vi "test_libssh2_hostkey_hash.vi"() -> ()   [LabVIEW 2017, in "integration_tests.lvlib"]
uses:
  integration_tests.lvlib
  libssh2/Host Key Hash Type.ctl
  support/support.lvlib
  libssh2/libssh2.lvlib
  <vilib>/PNR/Transparent Assertions/Transparent Assertions/Transparent Assertions.lvlib
panel:
  out "error out":errorcluster
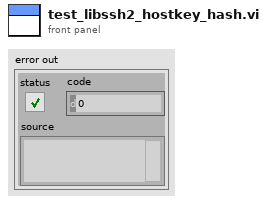
[diagram p1: front panel]
types:
  T1 = typedef "libssh2.lvlib/Host Key Hash Type.ctl" = enum16{"MD5", "SHA1", "SHA256"}
  T2 = typedef "libssh2.lvlib/Session Refnum.ctl" = refnum<k1>
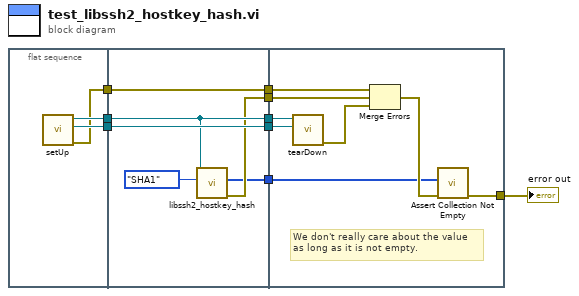
[diagram p0: block diagram]
diagram:
  n1 = flat-sequence {
    tunnel: [w12] -> w9
    tunnel: [w11] -> w8
    tunnel: [w10] -> w7
    tunnel: w9 -> [w15]
    tunnel: w8 -> [w18]
    tunnel: [w15] -> w6
    tunnel: [w18] -> w5
    tunnel: w7 -> [w17]
    tunnel: [w17] -> w4
    tunnel: [w14] -> w3
    tunnel: [w13] -> w2
    tunnel: w6 -> [w26]
    tunnel: w5 -> [w25]
    tunnel: [w24] -> w1
    tunnel: w4 -> [w22]
    tunnel: w3 -> [w20]
    tunnel: w2 -> [w19]
    frame #0 {
      n2 = call "setUp.vi"() -> ("error out"=w10:errorcluster, "connection ID"=w11:refnum<k5>, "session"=w12:T2)  [unwired: 9 in]
    }
    frame #1 {
      n3 = call "libssh2_hostkey_hash.vi"("hash type"=Host_Key_Hash_Type."SHA1", "session"=w15) -> ("error out"=w14:errorcluster, "hash"=w13:u8[])  [unwired: 8 in]
    }
    frame #2 {
      # "We don't really care about the value\nas long as it is not empty."
      n4 = call "tearDown.vi"("connection ID"=w25, "session"=w26) -> ("error out"=w23:errorcluster)  [unwired: 9 in]
      n5 = Merge Errors(w22, w20, w23) -> (w21:errorcluster)
      n6 = call <vilib>:"Assert Collection Not Empty.vi"("error in (no error)"=w21, "Collection"=w19) -> ("error out"=w24:errorcluster)  [unwired: 9 in]
    }
  }
  "error out" <- w1
